vi "CSM Example - Duplicate Modules.vi"() -> ()   [LabVIEW 2014]
uses:
  user.lib/_NEVSTOP/Communicable State Machine(CSM)/_Support/Priority Queue/Priority Queue.lvclass/Priority Queue.ctl
  user.lib/_NEVSTOP/Communicable State Machine(CSM)/Utility/uuid.vi
  user.lib/_NEVSTOP/Communicable State Machine(CSM)/_Support/Process/CSMP-Async Call.vi
  user.lib/_NEVSTOP/Communicable State Machine(CSM)/Utility/Trim Both Whitespace.vi
  user.lib/_NEVSTOP/Communicable State Machine(CSM)/_Support/CSMQ/_CSMObj-Message Check.vi
  user.lib/_NEVSTOP/Communicable State Machine(CSM)/_Support/CSMQ/_CSMObj-Enqueue Cross-Module Message.vi
  user.lib/_NEVSTOP/Communicable State Machine(CSM)/_Support/CSMQ/_CSMOFGV Get.vi
  user.lib/_NEVSTOP/Communicable State Machine(CSM)/_Support/Priority Queue/Enqueue Element.vi
  user.lib/_NEVSTOP/Communicable State Machine(CSM)/Utility/Build Error Cluster.vi
  user.lib/_NEVSTOP/Communicable State Machine(CSM)/_Support/CSMQ/_CSMOFGV.vi
  user.lib/_NEVSTOP/Communicable State Machine(CSM)/Communicable State Machine.lvlib
panel:
  out "Module Names":string[](array[string])
  in  "List Module":bool
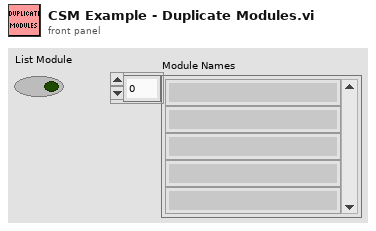
[diagram p1: front panel]
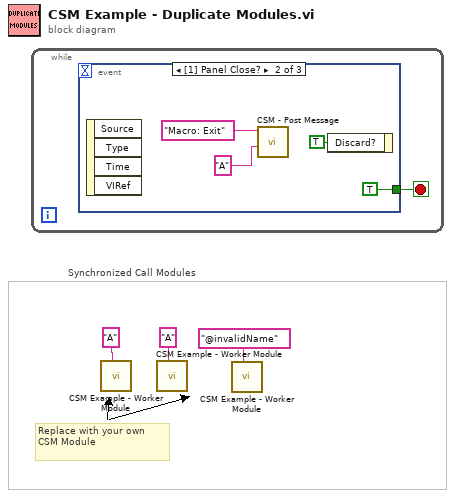
[diagram p0: block diagram]
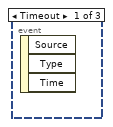
[diagram p2: hidden frame]
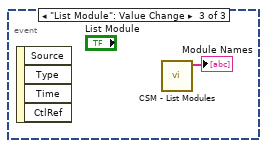
[diagram p3: hidden frame]
diagram:
  # "Replace with your own CSM Module"
  # "Synchronized Call Modules"
  n1 = while {
    stop <- w4 stop-if-true
    n2 = event shown="[1] Panel Close?" {
      selector: _ -> [_ _ _]
      dyn-events: _ -> [_ _ _]
      timeout: _ -> [_ _ _]
      tunnel: [_ TRUE ("Discard?") _] -> w4
      event Timeout {
        n3 = event-data() -> ()  [unwired: 1 in, 3 out]
      }
      event Panel Close? {
        n4 = event-data() -> ()  [unwired: 1 in, 4 out]
        n5 = call "CSM - Post Message.vi"("Target Module"="A" ("Name"), "State"="Macro: Exit" ("Name")) -> ()  [unwired: 9 in, 1 out]
        n6 = event-data("Discard?"=TRUE) -> ()  [unwired: 1 in, 1 out]
      }
      event "List Module": Value Change {
        n7 = event-data() -> ()  [unwired: 1 in, 4 out]
        n8 = call "CSM - List Modules.vi"() -> ("Module Names"=→"Module Names":string[])  [unwired: 10 in, 1 out]
      }
    }
  }
  n9 = call "CSM Example - Worker Module.vi"("Name(\"\" to use uuid)"="A" ("Name")) -> ()  [unwired: 11 in]
  n10 = call "CSM Example - Worker Module.vi"("Name(\"\" to use uuid)"="A" ("Name")) -> ()  [unwired: 11 in]
  n11 = call "CSM Example - Worker Module.vi"("Name(\"\" to use uuid)"="@invalidName" ("Name")) -> ()  [unwired: 11 in]
